vi "Teleop.vi"(10 "Match Info":T1={"Autonomous Elapsed Seconds"=0.0, "TeleOp Elapsed Seconds"=0.0, "Disabled Elapsed Seconds"=0.0, "Visited Autonomous"=FALSE, "Visited TeleOp"=FALSE, "Visited Disabled"=FALSE, "Autonomous Settings"={"Autonomous Style"=enum."Independent", "VI Refnum"=refnum}}, 11 "Call Context":T2) -> ()   [LabVIEW 2013]
doc: "This VI is called for each TeleOp packet received from the DS where the robot is not disabled. It is often used to read from the joysticks and update I/O or to update setpoints for timed control loops. It should complete and return within 20 milliseconds or it may miss DS packets."
uses:
  <vilib>/Rock Robotics/WPI/DriverStation/WPI_DriverStationDerivedRobotMode.ctl
  <vilib>/Rock Robotics/WPI/DriverStation/WPI_DriverStationMatch Info.ctl
  Robot Global Data.vi
  <vilib>/Rock Robotics/WPI/Joystick/WPI_JoystickGetSetRefNum.vi
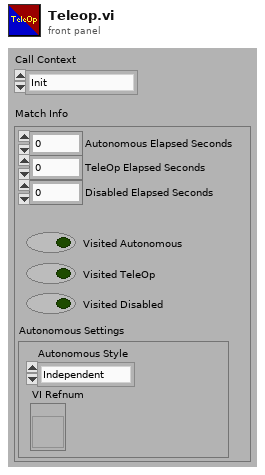
[diagram p1: front panel]
types:
  T1 = typedef "WPI_DriverStationMatch Info.ctl" = cluster{"Autonomous Elapsed Seconds":dbl, "TeleOp Elapsed Seconds":dbl, "Disabled Elapsed Seconds":dbl, "Visited Autonomous":bool, "Visited TeleOp":bool, "Visited Disabled":bool, "Autonomous Settings":cluster{"Autonomous Style":enum16{"Iterative", "Independent"}, "VI Refnum":refnum<vi>}}
  T2 = typedef "WPI_DriverStationDerivedRobotMode.ctl" = enum16{"Init", "Execute", "Stop"}
  T3 = typedef "WPI_JoystickDevRef.ctl" = cluster{"Device":T4}
  T4 = typedef "WPI_JoystickDeviceEnum.ctl" = enum16{"USB 1", "USB 2", "USB 3", "USB 4", "Kinect 1", "Kinect 2"}
  T5 = typedef "WPI_JoystickButtonState.ctl" = cluster{"Button 1":bool, "Button 2":bool, "Button 3":bool, "Button 4":bool, "Button 5":bool, "Button 6":bool, "Button 7":bool, "Button 8":bool, "Button 9":bool, "Button 10":bool, "Button 11":bool, "Button 12":bool}
  T6 = cluster{"axis 1 (x)":dbl, "axis 2 (y)":dbl, "axis 3 (throttle)":dbl, "axis 4":dbl, "axis 5":dbl, "axis 6":dbl}
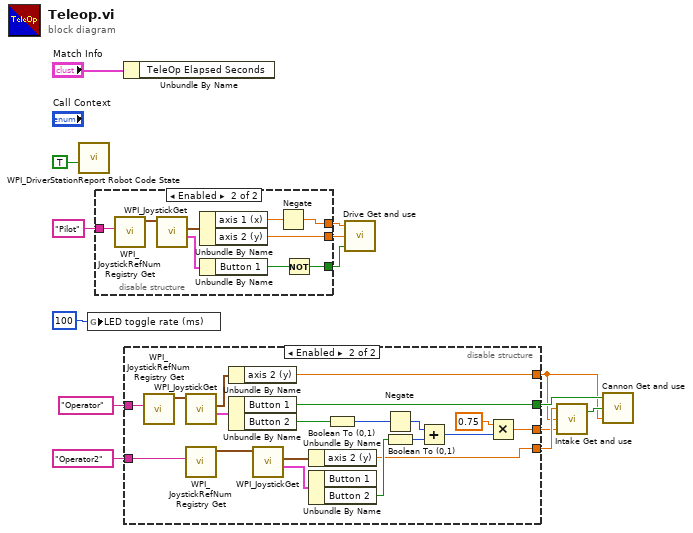
[diagram p0: block diagram]
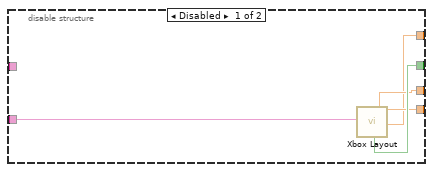
[diagram p2: hidden frame]
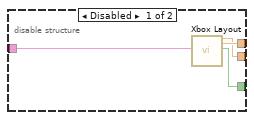
[diagram p3: hidden frame]
diagram:
  n1 = call <vilib>:"WPI_DriverStationReport Robot Code State.vi"("TeleOp"=TRUE ("Autonomous")) -> ()  [unwired: 10 in, 1 out]
  n2 = global write "Robot Global Data.vi" "LED toggle rate (ms)"(u32 100 ("LED ms toggle rate")) -> ()
  n3 = disable-structure shown="Enabled" {
    disable-tunnel: [w18 w21] -> w7
    disable-tunnel: [w17 w23] -> w6
    disable-tunnel: [w16 w19] -> w5
    disable-tunnel: "Pilot" ("refnum name") -> [w15 w27]
    frame Disabled {
      n4 = call "Xbox Layout.vi"("Joystick Name"=w15) -> ("Left Stick Y"=w17:dbl, "Left Stick X"=w18:dbl, "Left Stick Touch"=w16:bool)  [unwired: 3 in, 13 out]
    }
    frame Enabled {
      n5 = call <vilib>:"WPI_JoystickRefNum Registry Get.vi"("refnum name"=w27) -> ("JoystickDevRef"=w26:T3)  [unwired: 9 in, 1 out]
      n6 = call <vilib>:"WPI_JoystickGet.vi"("JoystickDevRef"=w26) -> ("Buttons"=w24:T5, "Axes"=w25:T6)  [unwired: 4 in, 1 out]
      n7 = Unbundle By Name(w25) -> ("axis 1 (x)"=w20:dbl, "axis 2 (y)"=w23:dbl)
      n8 = Unbundle By Name(w24) -> ("Button 1"=w22:bool)
      n9 = Negate(x=w20) -> (-x=w21:dbl)
      n10 = Not(x=w22) -> (.not. x?=w19:bool)
    }
  }
  n11 = Unbundle By Name("Match Info") -> ()  [unwired: 1 out]
  n12 = disable-structure shown="Enabled" {
    disable-tunnel: "Operator2" ("refnum name") -> [w32 w50]
    disable-tunnel: [w31 w35] -> w10
    disable-tunnel: [w30 w34] -> w9
    disable-tunnel: [w29 w42] -> w8
    disable-tunnel: [w28 w33] -> w2
    disable-tunnel: "Operator" ("refnum name") -> [_ w41]
    frame Disabled {
      n13 = call "Xbox Layout.vi"("Joystick Name"=w32) -> ("X"=w31:bool, "L+R Throttles"=w29:dbl, "Left Stick Y"=w30:dbl, "Right Stick Y"=w28:dbl)  [unwired: 3 in, 12 out]
    }
    frame Enabled {
      n14 = call <vilib>:"WPI_JoystickRefNum Registry Get.vi"("refnum name"=w41) -> ("JoystickDevRef"=w40:T3)  [unwired: 9 in, 1 out]
      n15 = call <vilib>:"WPI_JoystickGet.vi"("JoystickDevRef"=w40) -> ("Buttons"=w38:T5, "Axes"=w39:T6)  [unwired: 4 in, 1 out]
      n16 = call <vilib>:"WPI_JoystickRefNum Registry Get.vi"("refnum name"=w50) -> ("JoystickDevRef"=w51:T3)  [unwired: 9 in, 1 out]
      n17 = Unbundle By Name(w39) -> ("axis 2 (y)"=w33:dbl)
      n18 = Unbundle By Name(w38) -> ("Button 1"=w35:bool, "Button 2"=w37:bool)
      n19 = call <vilib>:"WPI_JoystickGet.vi"("JoystickDevRef"=w51) -> ("Buttons"=w48:T5, "Axes"=w49:T6)  [unwired: 4 in, 1 out]
      n20 = Unbundle By Name(w49) -> ("axis 2 (y)"=w34:dbl)
      n21 = Unbundle By Name(w48) -> ("Button 2"=w36:bool)  [unwired: 1 out]
      n22 = Boolean To (0,1)(Boolean=w37) -> (0, 1=w43:i16)
      n23 = Negate(x=w43) -> (-x=w44:i16)
      n24 = Boolean To (0,1)(Boolean=w36) -> (0, 1=w45:i16)
      n25 = Add(x=w44, y=w45) -> (x+y=w47:i16)
      n26 = Multiply(x=0.75, y=w47) -> (x*y=w42:dbl)
    }
  }
  n27 = call "Drive Get and use.vi"("Slow Drive"=w5, "Y - Axis"=w6, "X - Axis"=w7) -> ()
  n28 = call "Intake Get and use.vi"("TakeBall"=w8, "Cannon vbus"=w2, "Upper Claw"=w9) -> ("InTake Max"=w4:bool)  [unwired: 1 out]
  n29 = call "Cannon Get and use.vi"("Move"=w2, "InTake Max"=w4, "Fire"=w10) -> ()  [unwired: 1 out]
